vi "ArrayUnbundler.vi"(1 "Array":cluster{"Array":dbl[]}[](array[cluster])) -> (0 "Array 2":dbl[](array[numeric]))   [LabVIEW 2015]
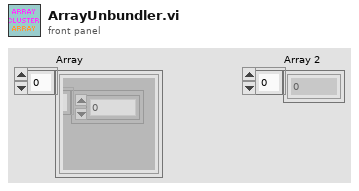
[diagram p1: front panel]
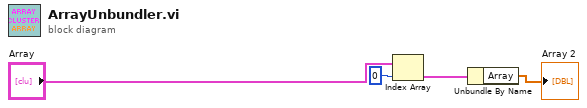
[diagram p0: block diagram]
diagram:
  n1 = Index Array(array="Array", index=0) -> (element=w3:cluster{"Array":dbl[]})
  n2 = Unbundle By Name(w3) -> ("Array"=→"Array 2":dbl[])
